vi "Example - SLL Database.vi"() -> ()   [LabVIEW 2014, in "SLL Database.lvclass"]
uses:
  SLL Database.lvclass
panel:
  out "Data Output":string[][](array[string])=[["1"]]
  in  "Query":string="SELECT 1"
  in  "Database Connection":T1={"Database Driver"="PostgreSQL Unicode", "Server"="127.0.0.1", "Port"=5432, "Database"="postgres", "User ID"="postgres", "Password"="postgres"}
  out "error out":errorcluster
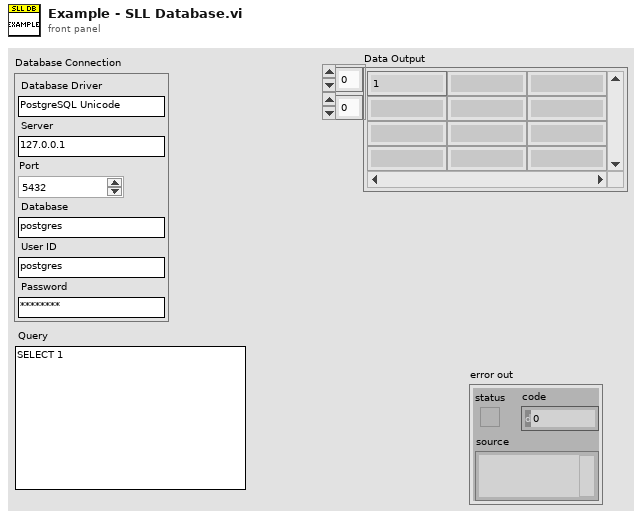
[diagram p1: front panel]
types:
  T1 = cluster{"Database Driver":string, "Server":string, "Port":i32, "Database":string, "User ID":string, "Password":string}
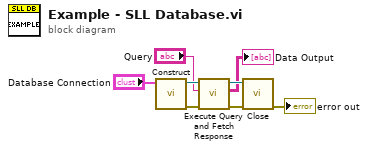
[diagram p0: block diagram]
diagram:
  n1 = call "Construct.vi"("Database Connection"="Database Connection") -> ("error out"=w6:errorcluster, "SLL Database out"=w8:refnum<class "SLL Database.lvclass">)  [unwired: 9 in]
  n2 = call "Execute Query and Fetch Response.vi"("error in (no error)"=w6, "Query"="Query", "SLL Database in"=w8) -> ("error out"=w5:errorcluster, "Data Output"=→"Data Output":string[][], "SLL Database out"=w7:refnum<class "SLL Database.lvclass">)  [unwired: 6 in]
  n3 = call "Close.vi"("error in (no error)"=w5, "SLL Database in"=w7) -> ("error out"=→"error out":errorcluster)  [unwired: 8 in, 1 out]
